vi "DeleteFrame.vi"(8 "error in (no error)":errorcluster, 10 "Frame Index":u32, 11 "FrameSlot_Root in":refnum<class "FrameSlot_Root.lvclass">) -> (0 "error out":errorcluster, 3 "FrameSlot_Root out":refnum<class "FrameSlot_Root.lvclass">)   [LabVIEW 2018, in "FrameSlot_Root.lvclass"]
uses:
  FrameSlot_Root.lvclass
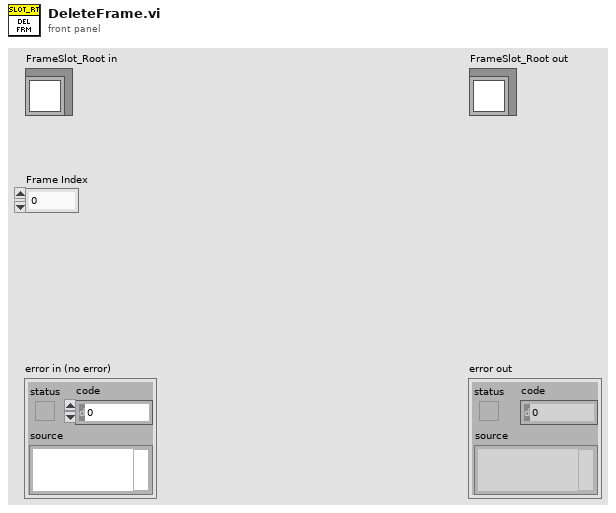
[diagram p1: front panel]
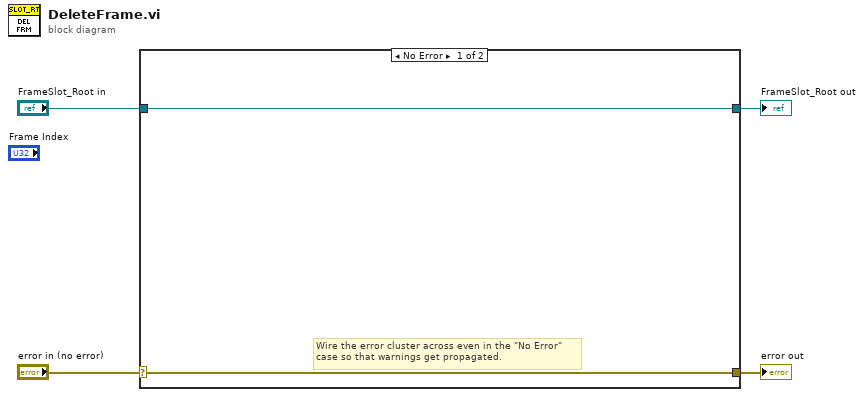
[diagram p0: block diagram]
diagram:
  n1 = case shown="No Error" "error in (no error)" {
    selector: "error in (no error)" -> [w5 w8]
    tunnel: [w5 w8] -> w3
    tunnel: [w6 w7] -> w1
    tunnel: "FrameSlot_Root in" -> [w6 w7]
    frame No Error {
      # "Wire the error cluster across even in the \"No Error\"\ncase so that warnings get propagated."
    }
    frame Error {
    }
  }
  "error out" <- w3
  "FrameSlot_Root out" <- w1
